vi "Connect.vi"(8 "error in (no error)":errorcluster, 11 "Motion in":refnum<class "Motion.lvclass">) -> (0 "error out":errorcluster, 3 "Motion out":refnum<class "Motion.lvclass">)   [LabVIEW 2020, in "Motion.lvclass"]
uses:
  Motion.lvclass
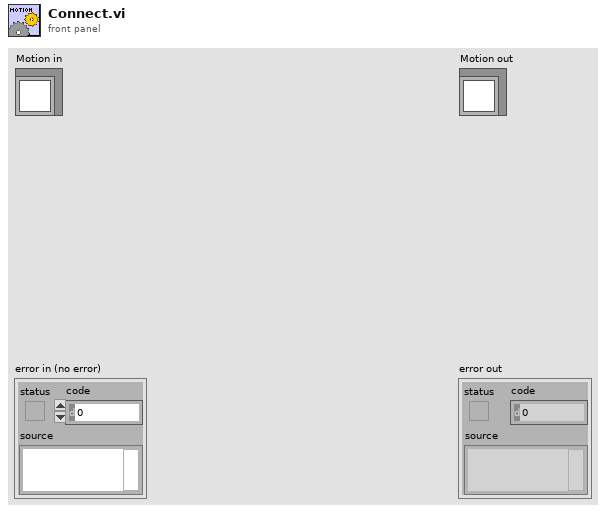
[diagram p1: front panel]
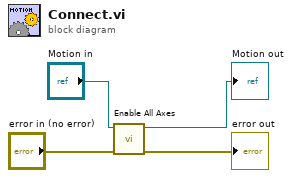
[diagram p0: block diagram]
diagram:
  n1 = call-dynamic "Enable All Axes.vi"("error in (no error)"="error in (no error)", "Motion in"="Motion in") -> ("error out"=→"error out":errorcluster, "Motion out"=→"Motion out":refnum<class "Motion.lvclass">)  [unwired: 8 in]
